vi "czujki.vi"(7 "LabVIEW Web Service Request":refnum<class "Web Request.lvclass">) -> (1 "time_stemp":string, 2 "sensors":string)   [LabVIEW 2024]
uses:
  <vilib>/wsapi/Web Request.lvclass
panel:
  # "Each additional control wired to the connector pane will be available as an input in the URL. To include an indicator in terminal-mode output (the default setting), it must also be wired to the connector pane."
  # "Use the Web Service Request input terminal to call the VIs on the Web Services palette. Do not remove it from the connector pane unless you don't need access to the palette."
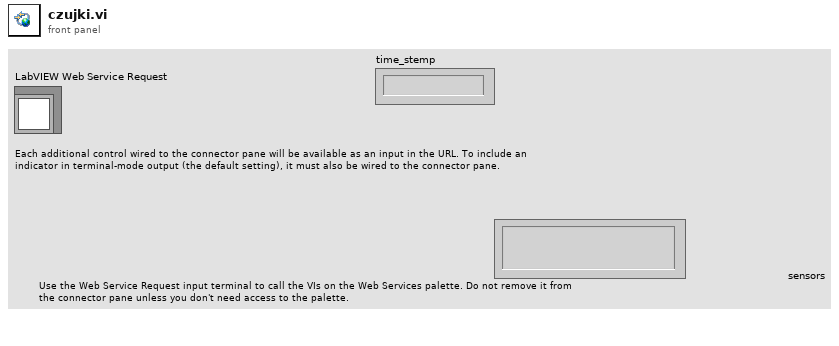
[diagram p1: front panel]
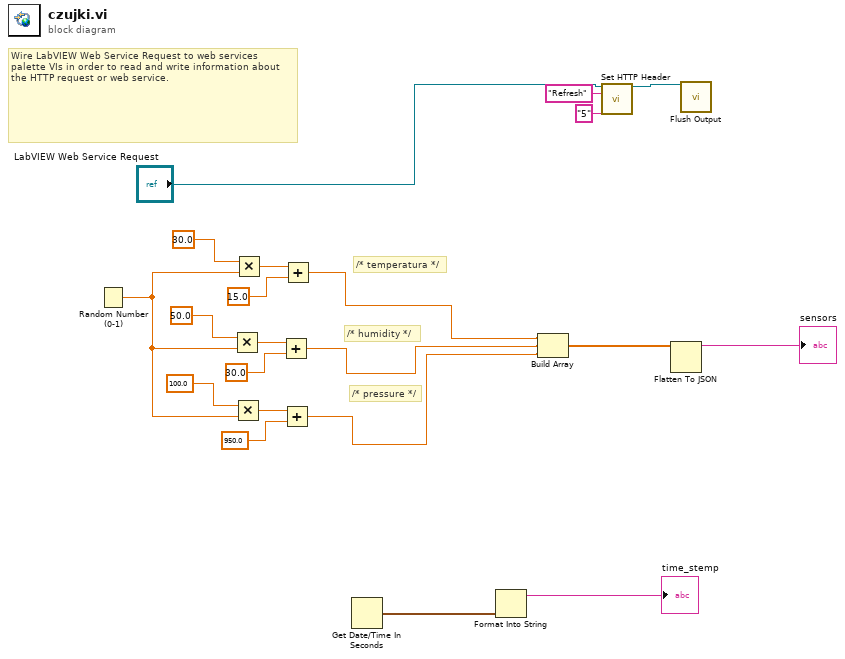
[diagram p0: block diagram]
diagram:
  # "/* pressure */"
  # "/* humidity */"
  # "/* temperatura */"
  # "Wire LabVIEW Web Service Request to web services palette VIs in order to read and write information about the HTTP request or web service."
  n1 = Random Number (0-1)() -> (number: 0 to 1=w12:dbl)
  n2 = Multiply(x=50.0, y=w12) -> (x*y=w17:dbl)
  n3 = Multiply(x=100.0, y=w12) -> (x*y=w14:dbl)
  n4 = Multiply(x=30.0, y=w12) -> (x*y=w20:dbl)
  n5 = Add(x=w17, y=30.0) -> (x+y=w10:dbl)
  n6 = Add(x=w14, y=950.0) -> (x+y=w9:dbl)
  n7 = Add(x=w20, y=15.0) -> (x+y=w11:dbl)
  n8 = Get Date/Time In Seconds() -> (seconds since 1Jan1904=w2:timestamp)
  n9 = Format Into String(w2) -> (resulting string=→"time_stemp":string)  [unwired: 3 in, 1 out]
  n10 = Build Array(w11, w10, w9) -> (w8:dbl[])
  n11 = call <vilib>:"Set HTTP Header.vi"("LabVIEW Web Service Request"="LabVIEW Web Service Request", "header"="Refresh", "header value"="5") -> ("LabVIEW Web Service Request out"=w4:refnum<class "Web Request.lvclass">)  [unwired: 11 in, 1 out]
  n12 = Flatten To JSON(anything=w8) -> (JSON string=→"sensors":string)  [unwired: 2 in, 1 out]
  n13 = call <vilib>:"Flush Output.vi"("LabVIEW Web Service Request"=w4) -> ()  [unwired: 13 in, 2 out]
